vi "VersionTokens.vi"() -> (3 "Array":string[](array[string]))   [LabVIEW 2019, in "ByteLVDevEnv.lvlib"]
uses:
  ByteLVDevEnv.lvlib
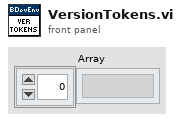
[diagram p1: front panel]
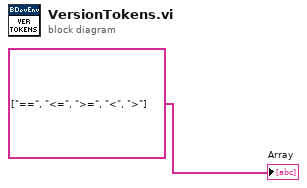
[diagram p0: block diagram]
diagram:
  "Array" <- string[] ["==", "<=", ">=", "<", ">"]
